vi "TableReady.vi"(0 "VISA resource name":refnum<visa-resource-name>) -> (4 "VISA resource name dup":refnum<visa-resource-name>, 8 "Ready ?":bool, 15 "Error Out":errorcluster)   [LabVIEW 2011]
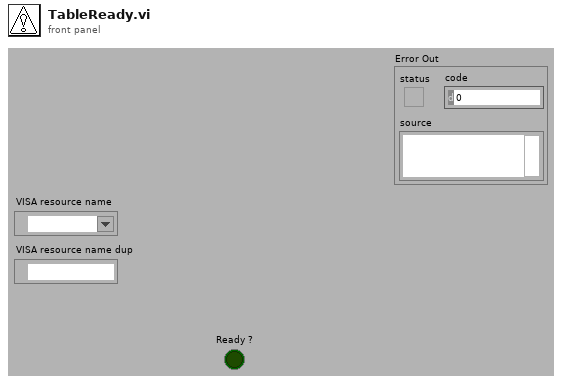
[diagram p1: front panel]
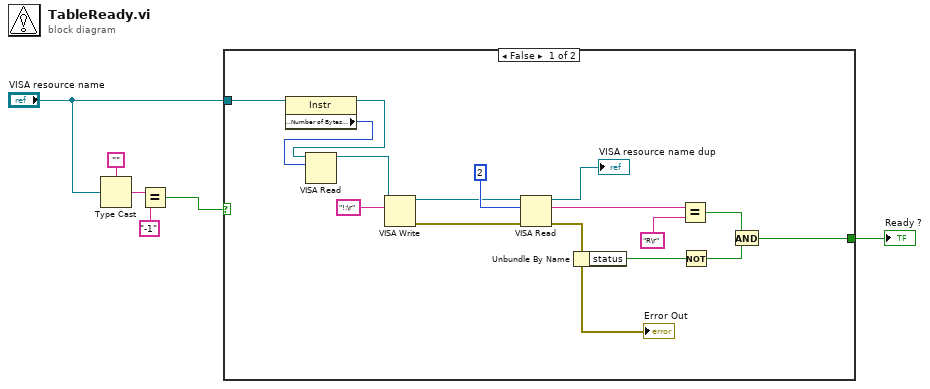
[diagram p0: block diagram]
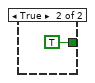
[diagram p2: hidden frame]
diagram:
  n1 = Type Cast(type="", x="VISA resource name") -> (*(type *) &x=w4:string)
  n2 = Equal?(x=w4, y="-1") -> (x = y?=w2:bool)
  n3 = case shown="False" w2 {
    tunnel: [w20 TRUE] -> w6
    tunnel: "VISA resource name" -> [w11 _]
    frame False {
      n4 = property class="Instr"(reference=w11) -> (reference out=w9:refnum<visa-resource-name>, "Serial Settings:Number of Bytes at Serial Port"=w10:u32)  [unwired: 1 in, 1 out]
      n5 = VISA Read(VISA resource name=w9, byte count=w10) -> (VISA resource name out=w8:refnum<visa-resource-name>)  [unwired: 1 in, 3 out]
      n6 = VISA Write(VISA resource name=w8, write buffer="!:\r") -> (VISA resource name out=w13:refnum<visa-resource-name>, error out=w15:errorcluster)  [unwired: 1 in, 1 out]
      n7 = VISA Read(VISA resource name=w13, byte count=u32 2, error in (no error)=w15) -> (VISA resource name out=→"VISA resource name dup":refnum<visa-resource-name>, read buffer=w22:string, error out=w7:errorcluster)  [unwired: 1 out]
      "Error Out" <- w7
      n8 = Unbundle By Name(w7) -> ("status"=w18:bool)
      n9 = Equal?(x=w22, y="R\r") -> (x = y?=w19:bool)
      n10 = Not(x=w18) -> (.not. x?=w17:bool)
      n11 = And(x=w19, y=w17) -> (x .and. y?=w20:bool)
    }
    frame True {
    }
  }
  "Ready ?" <- w6
